vi "DataTypes.vi"() -> ()   [LabVIEW 2020]
panel:
  out "Boolean 2":bool
  in  "var4":bool
  out "var3 2":string
  in  "var3":string
  out "var2 2":u8
  in  "var2":u8
  out "var1 2":dbl
  in  "var1":dbl
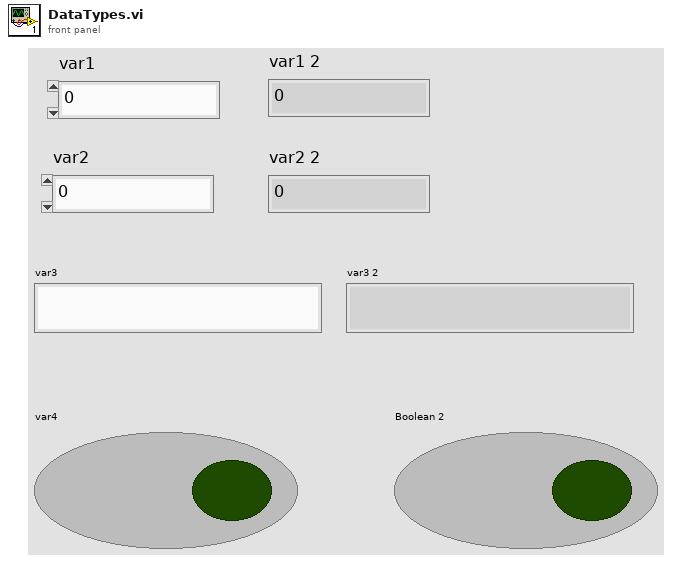
[diagram p1: front panel]
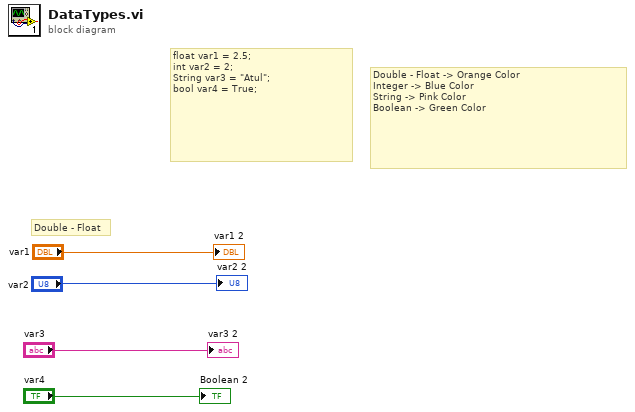
[diagram p0: block diagram]
diagram:
  # "Double - Float -> Orange Color\nInteger -> Blue Color\nString -> Pink Color\nBoolean -> Green Color"
  # "Double - Float"
  # "float var1 = 2.5;\nint var2 = 2;\nString var3 = \"Atul\";\nbool var4 = True;"
  "var1 2" <- "var1"
  "var2 2" <- "var2"
  "var3 2" <- "var3"
  "Boolean 2" <- "var4"
